vi "L298N_Driver.vi"() -> ()   [LabVIEW 2019]
uses:
  Commande 2.ctl
  <vilib>/myRIO/Instrument Drivers/Onboard IO/DIO/typedefs/DIO Reference.ctl
  <vilib>/myRIO/Common/Instrument Driver Framework/Utilities/typedefs/myRIO Generic Hardware Reference.ctl
  <vilib>/myRIO/Common/Instrument Driver Framework/Utilities/typedefs/Hardware Version Enum.ctl
  <vilib>/myRIO/Common/Instrument Driver Framework/Utilities/typedefs/myRIO v1.0 Reference.ctl
  <vilib>/myRIO/Common/Instrument Driver Framework/Utilities/typedefs/Generic FPGA Reference.ctl
  <vilib>/myRIO/Common/Instrument Driver Framework/myRIO v1.0/DIO/typedefs/DIO Channels List.ctl
  <vilib>/myRIO/Common/Instrument Driver Framework/myRIO v1.0/DIO/typedefs/DIO Channels Enum.ctl
  <vilib>/userDefined/High Color/nirio_resource_hc.ctl
  <vilib>/myRIO/Common/Instrument Driver Framework/myRIO v1.0/DIO/vis/myRIO v1.1 Open DIO.vi
  <vilib>/myRIO/Common/Instrument Driver Framework/Utilities/vis/Validate Channels.vi
  <vilib>/myRIO/Common/Instrument Driver Framework/myRIO v1.0/DIO/vis/myRIO v1.0 Reserve DIO.vi
  <vilib>/myRIO/Common/Instrument Driver Framework/myRIO v1.0/DIO/vis/myRIO v1.0 Close DIO.vi
  <vilib>/myRIO/Common/Instrument Driver Framework/myRIO v1.0/Resource Manager/vis/myRIO v1.0 Reserve Channel List.vi
  <vilib>/myRIO/Common/Instrument Driver Framework/myRIO v1.0/DIO/vis/myRIO v1.0 Build MUX Configuration DIO.vi
  <vilib>/myRIO/Common/Instrument Driver Framework/myRIO v1.0/DIO/vis/myRIO v1.0 Unreserve DIO.vi
  <vilib>/myRIO/Common/Instrument Driver Framework/myRIO v1.0/Resource Manager/vis/myRIO v1.0 Reserve Channel.vi
  <vilib>/myRIO/Common/Instrument Driver Framework/myRIO v1.0/Resource Manager/vis/myRIO v1.0 Unreserve Channel.vi
  <vilib>/myRIO/Common/Instrument Driver Framework/myRIO v1.0/Resource Manager/vis/myRIO v1.0 Create Configuration List.vi
  <vilib>/myRIO/Common/Instrument Driver Framework/myRIO v1.0/Resource Manager/vis/myRIO v1.0 Unreserve Channel List.vi
  <vilib>/myRIO/Common/Instrument Driver Framework/myRIO v1.0/Resource Manager/vis/myRIO v1.0 Build Mutex Name.vi
  <vilib>/Utility/VariantDataType/GetNumericInfo.vi
  <vilib>/Utility/error.llb/Error Cluster From Error Code.vi
  <vilib>/myRIO/Common/Instrument Driver Framework/myRIO v1.0/myRIO v1.1 Open.vi
  <vilib>/myRIO/Common/Instrument Driver Framework/Utilities/vis/IO Manager.vi
  <vilib>/myRIO/Common/Instrument Driver Framework/Utilities/vis/Configuration Manager.vi
  <vilib>/myRIO/Common/Instrument Driver Framework/myRIO v1.0/Resource Manager/vis/myRIO v1.0 Configure IO.vi
  <vilib>/myRIO/Common/Instrument Driver Framework/myRIO v1.0/myRIO v1.0 Close.vi
  <vilib>/myRIO/Common/Instrument Driver Framework/myRIO v1.0/DIO/vis/myRIO v1.0 Write DIO.vi
  <vilib>/myRIO/Common/Instrument Driver Framework/myRIO v1.0/DIO/vis/myRIO v1.0 Shutdown DIO.vi
  <vilib>/myRIO/Instrument Drivers/Onboard IO/DIO/vis/myRIO DIO Open.xnode
  <vilib>/myRIO/Instrument Drivers/Onboard IO/DIO/DIO.lvlib
panel:
  in  "Bouton Stop":bool
  out "Var_Etat":T1
  in  "PF_0":bool
  in  "PF_3":bool
  in  "PF_2":bool
  in  "PF_1":bool
  in  "PO_0":bool
  in  "PO_3":bool
  in  "PO_2":bool
  in  "PO_1":bool
  out "Moteur Porte 3":bool
  out "Moteur Porte 2":bool
  out "Moteur Porte 1":bool
  out "Moteur Porte 0":bool
  out "Moteur Cabine":bool
  in  "P0":bool
  in  "P3":bool
  in  "P2":bool
  in  "P1":bool
  in  "Etat_Asc":T1
  in  "Dest_3":bool
  in  "Dest_2":bool
  in  "Dest_1":bool
  in  "Dest_0":bool
  in  "Appel_0":bool
  in  "Appel_3":bool
  in  "Appel_2":bool
  in  "Appel_1":bool
  out "Cluster":T2
  in  "Énum":T3(ring)
  out "Etat":string
  out "Etat Ouvrir Porte 1":bool
  in  "Ouvrir Porte 1":bool
  out "error out 4":errorcluster caption="error out"
  in  "error in (no error) 4":errorcluster caption="error in (no error)"
  in  "Fermer  Porte 1":bool
  out "error out 3":errorcluster caption="error out"
  in  "error in (no error) 3":errorcluster caption="error in (no error)"
  out "error out 2":errorcluster caption="error out"
  in  "error in (no error) 2":errorcluster caption="error in (no error)"
  in  "Cabine Descendre":bool
  out "error out":errorcluster
  in  "error in (no error)":errorcluster
  in  "Cabine Monter":bool
  # "Simulation de présence cabine"
  # "Simulation de portes"
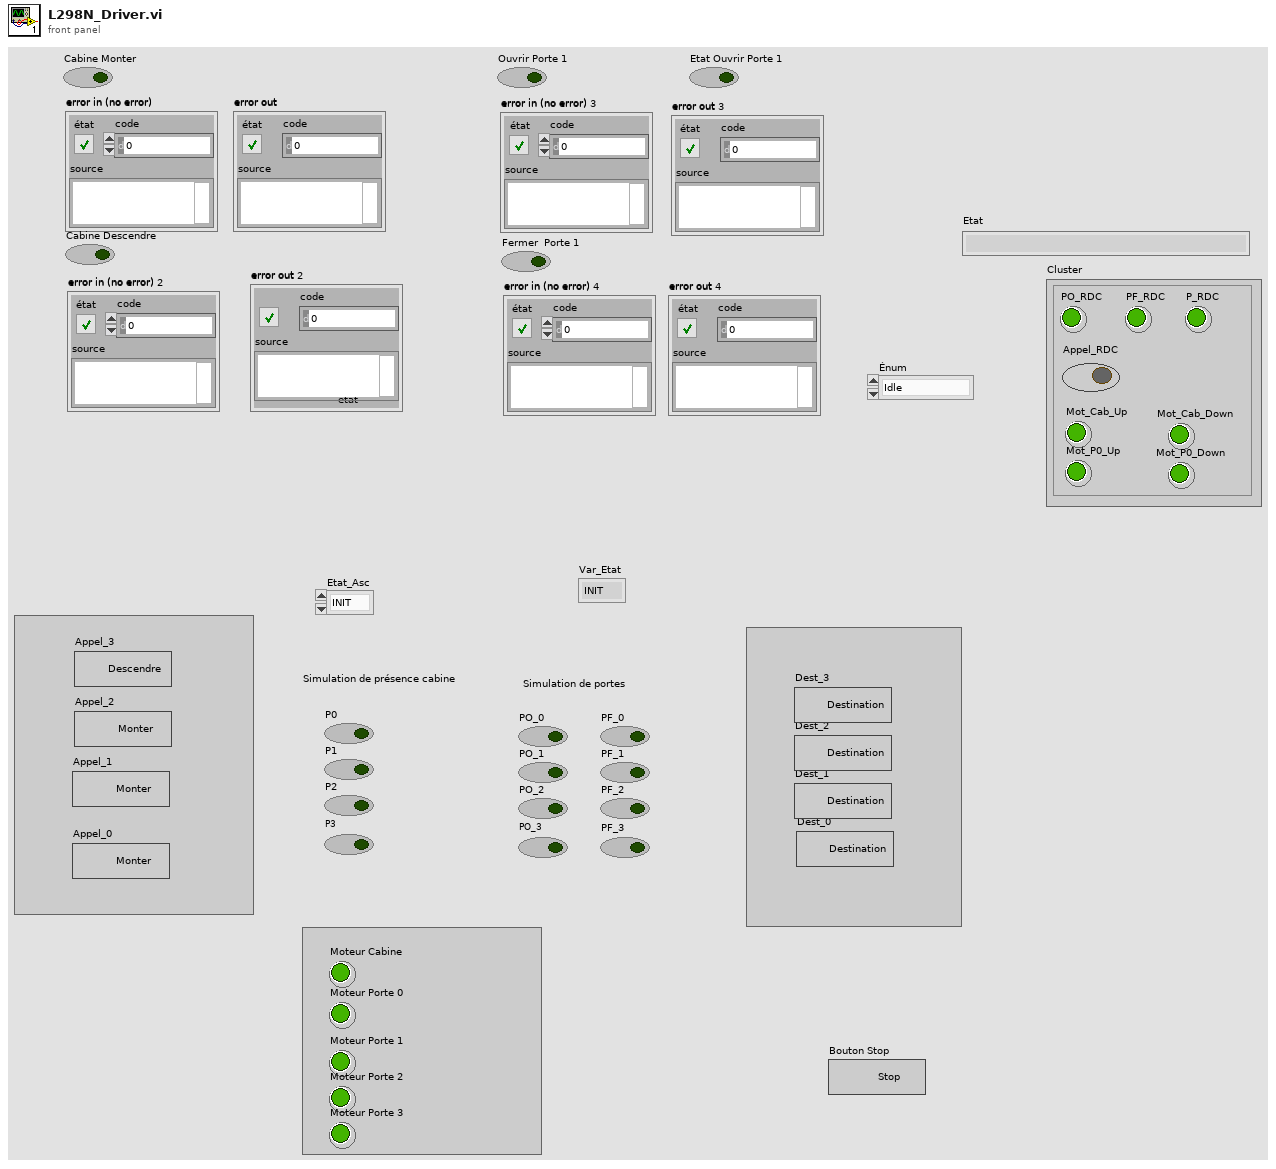
[diagram p1: front panel]
types:
  T1 = typedef "Commande 2.ctl" = enum16{"INIT", "REPOS", "DEPLACEMENT", "OUVERTURE_PORTE", "ATTENTE_TEMPO", "FERMETURE_PORTE", "ARRET_URGENCE"}
  T2 = cluster{"PO_RDC":bool, "PF_RDC":bool, "P_RDC":bool, "Appel_RDC":bool, "Mot_Cab_Up":bool, "Mot_Cab_Down":bool, "Mot_P0_Up":bool, "Mot_P0_Down":bool}
  T3 = enum16{"Idle", "Appel_Etage0", "Descente_Cabine", "Arrivee_Etage0", "Ouverture_Porte", "Attente_Porte", "Fermerture_Porte", "Fin", ""}
  T4 = typedef "DIO.lvlib/DIO Reference.ctl" = cluster{"myRIO Reference":T5, "DIO Channels List":T9}
  T5 = typedef "myRIO Generic Hardware Reference.ctl" = cluster{"myRIO Model":T6, "myRIO Hardware Reference":T7}
  T6 = typedef "Hardware Version Enum.ctl" = enum16{"Unknown", "myRIO-1900", "myRIO-1950", "roboRIO", "NI ELVIS RIO CM", "ELVIS III"}
  T7 = typedef "myRIO v1.0 Reference.ctl" = cluster{"Generic FPGA Reference":T8, "Allow multiple opens":bool}
  T8 = typedef "Generic FPGA Reference.ctl" = refnum<k20>
  T9 = typedef "DIO Channels List.ctl" = T10[]
  T10 = typedef "DIO Channels Enum.ctl" = enum16{"Not Connected", "C/DIO0", "C/DIO1", "C/DIO2", "C/DIO3", "C/DIO4", "C/DIO5", "C/DIO6", "C/DIO7", "A/DIO0", "A/DIO1", "A/DIO2", "A/DIO3", "A/DIO4", "A/DIO5", "A/DIO6", "A/DIO7", "A/DIO8", "A/DIO9", "A/DIO10", "A/DIO11", "A/DIO12", "A/DIO13", "A/DIO14", "A/DIO15", "A/DIO16", "A/DIO17", "A/DIO18", "A/DIO19", "B/DIO0", "B/DIO1", "B/DIO2", "B/DIO3", "B/DIO4", "B/DIO5", "B/DIO6", "B/DIO7", "B/DIO8", "B/DIO9", "B/DIO10", "B/DIO11", "B/DIO12", "B/DIO13", "B/DIO14", "B/DIO15", "B/DIO16", "B/DIO17", "B/DIO18", "B/DIO19", "LED0", "LED1", "LED2", "LED3", "Button0", "DIO/DIO0", "DIO/DIO1", "DIO/DIO2", "DIO/DIO3", "DIO/DIO4", "DIO/DIO5", "DIO/DIO6", "DIO/DIO7", "DIO/DIO8", "DIO/DIO9", "SPI/CS0", "SPI/CS1", "SPI/CS2", "SPI/CS3", "LED RADIO (Green)", "LED RADIO (Red)", "LED COMM (Green)", "LED COMM (Red)", "LED MODE (Green)", "LED MODE (Red)"}
  T11 = typedef "nirio_resource_hc.ctl" = tag
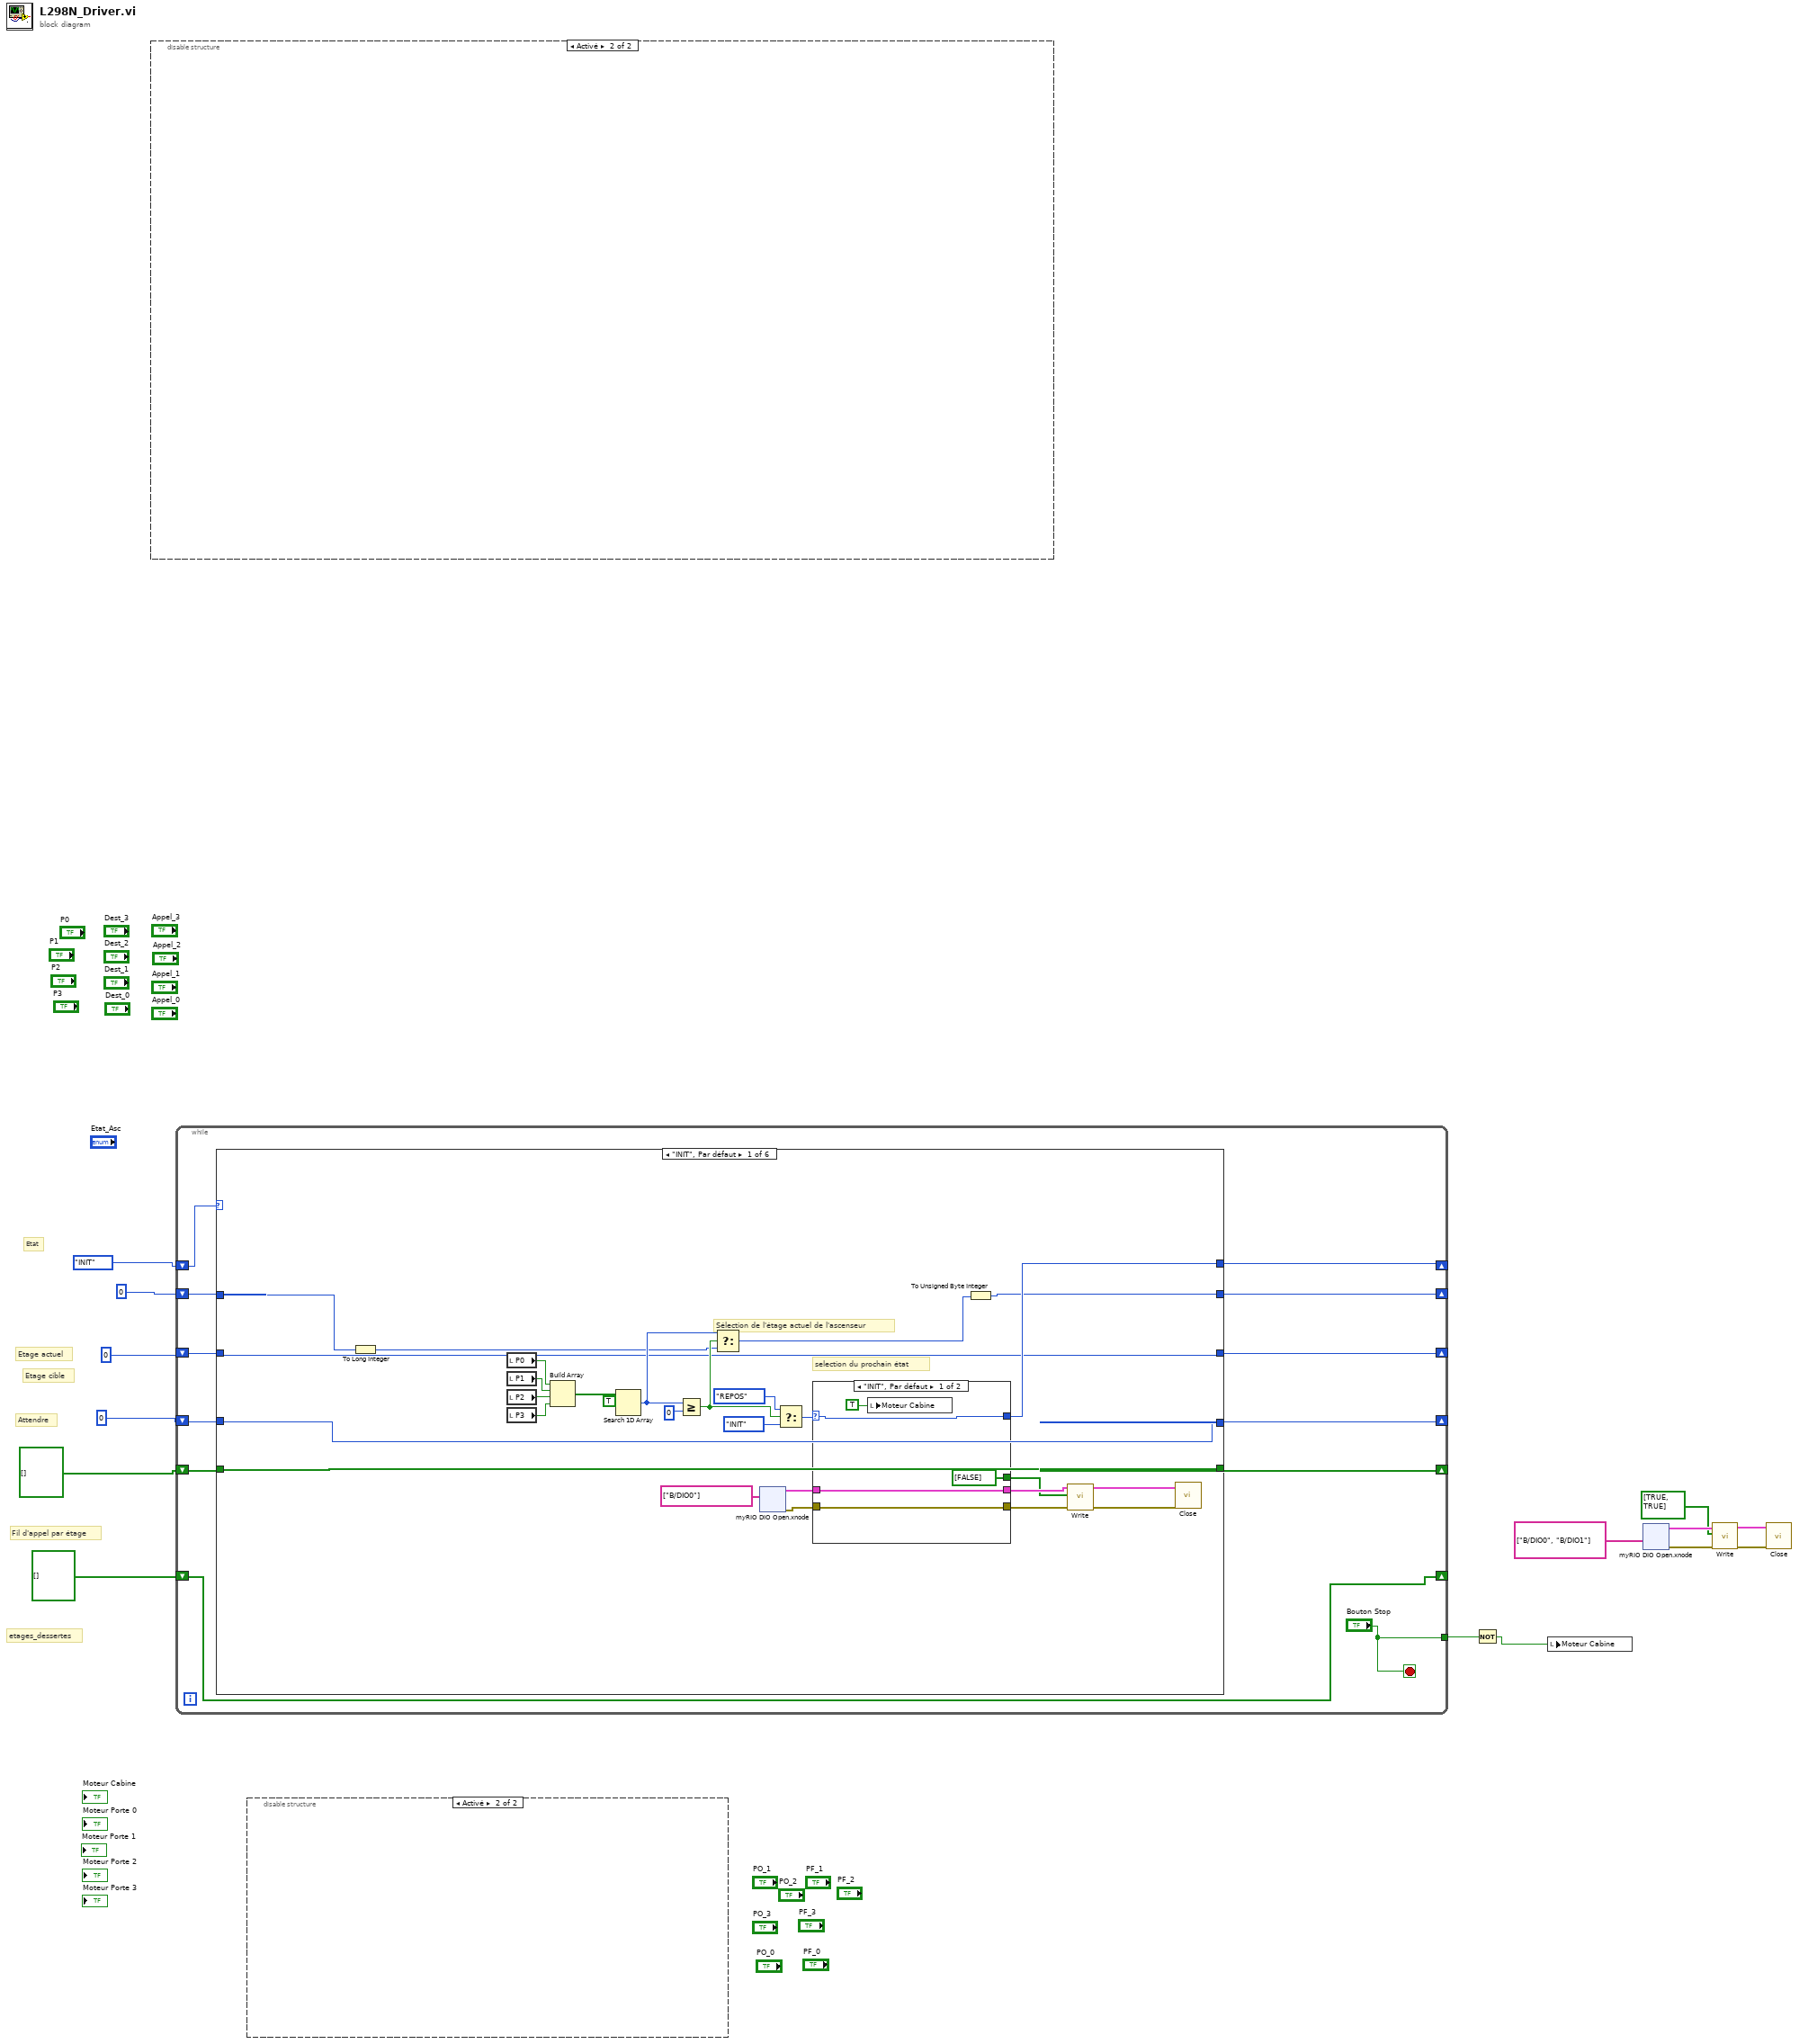
[diagram p0: block diagram]
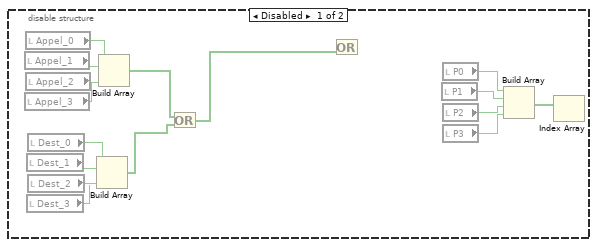
[diagram p2: hidden frame]
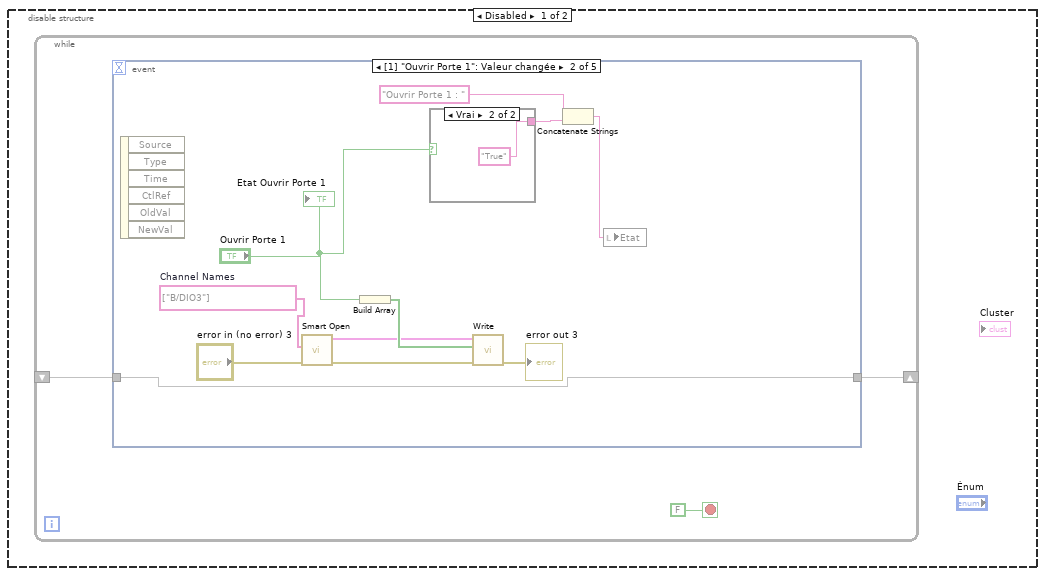
[diagram p3: hidden frame]
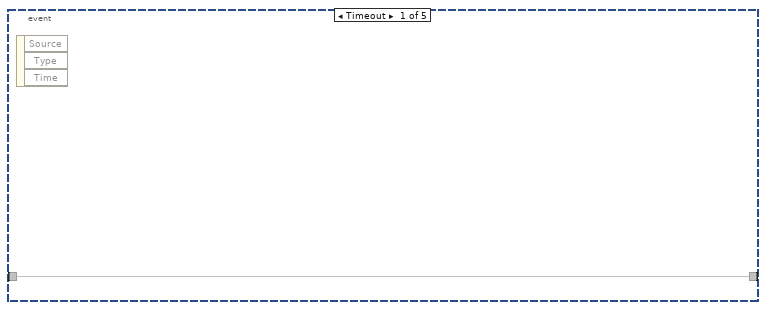
[diagram p4: hidden frame]
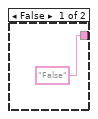
[diagram p5: hidden frame]
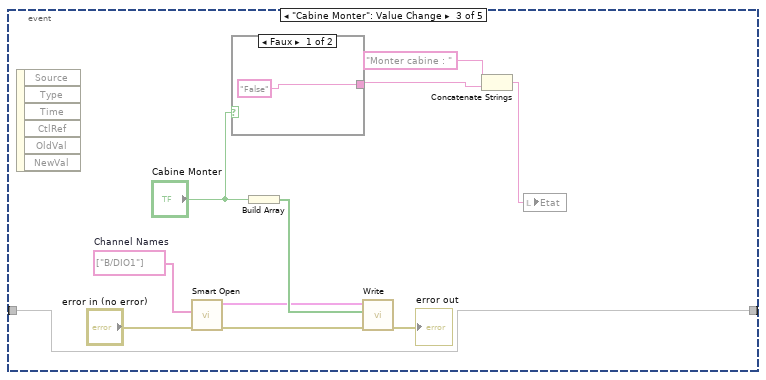
[diagram p6: hidden frame]
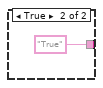
[diagram p7: hidden frame]
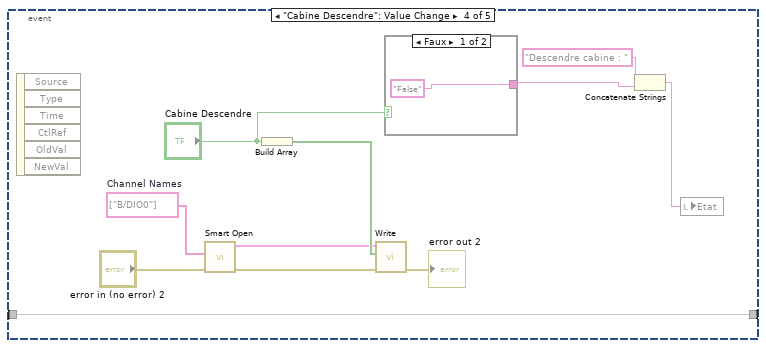
[diagram p8: hidden frame]
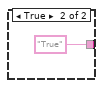
[diagram p9: hidden frame]
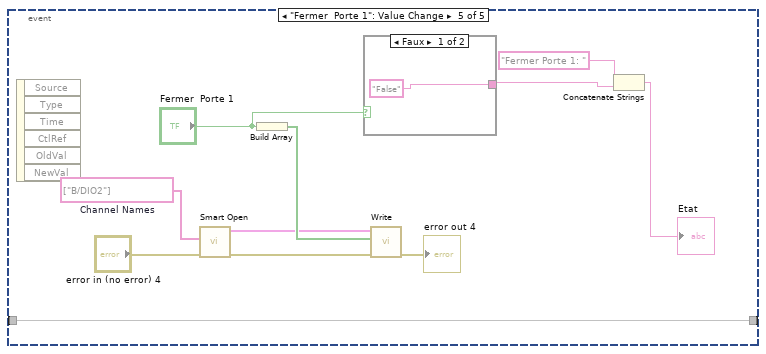
[diagram p10: hidden frame]
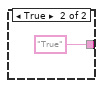
[diagram p11: hidden frame]
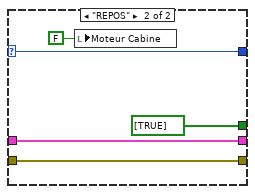
[diagram p12: hidden frame]
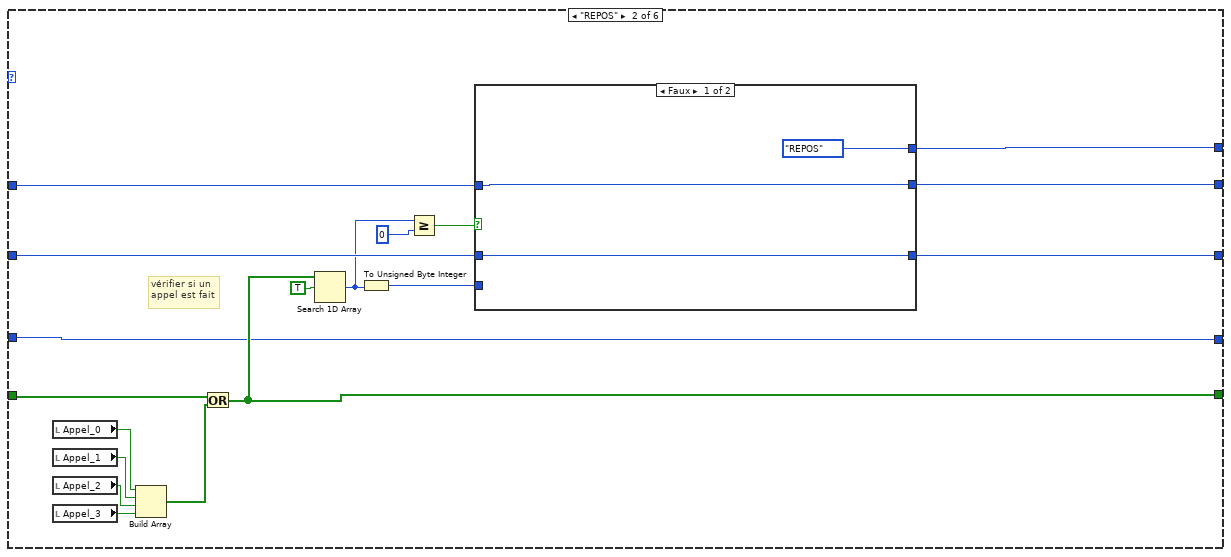
[diagram p13: hidden frame]
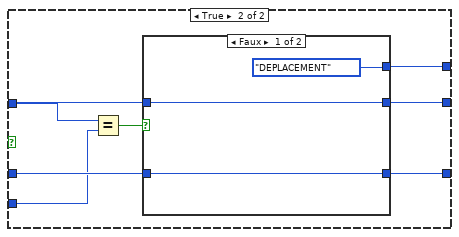
[diagram p14: hidden frame]
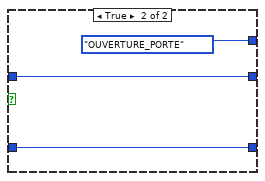
[diagram p15: hidden frame]
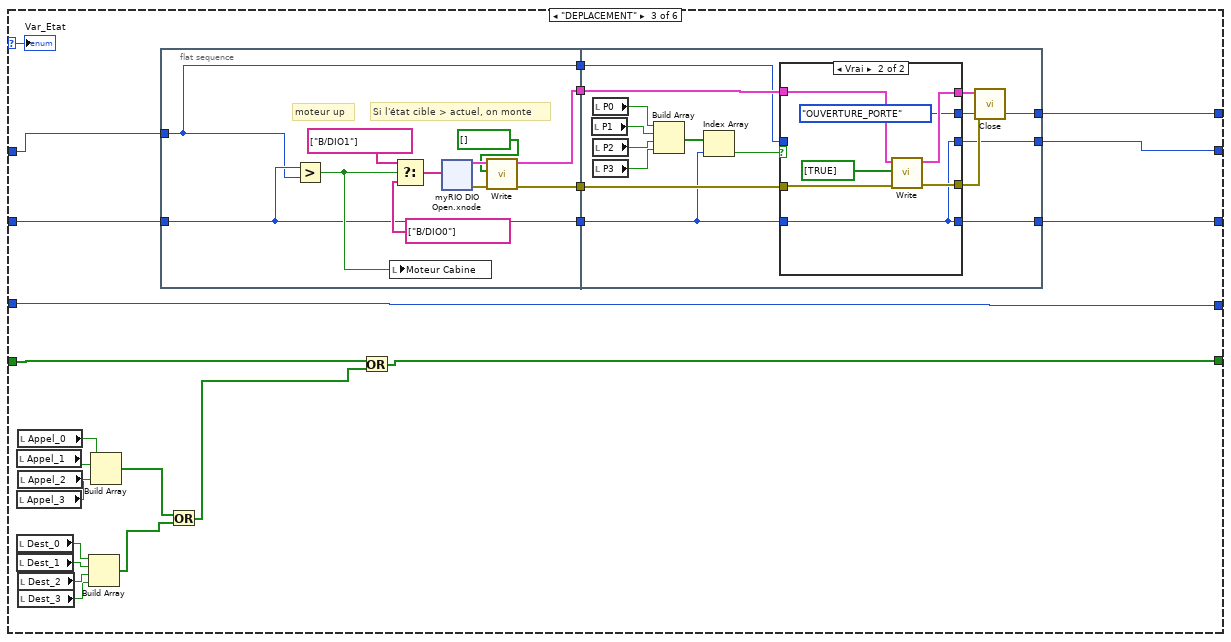
[diagram p16: hidden frame]
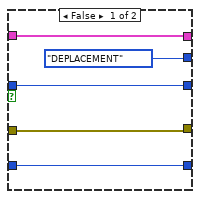
[diagram p17: hidden frame]
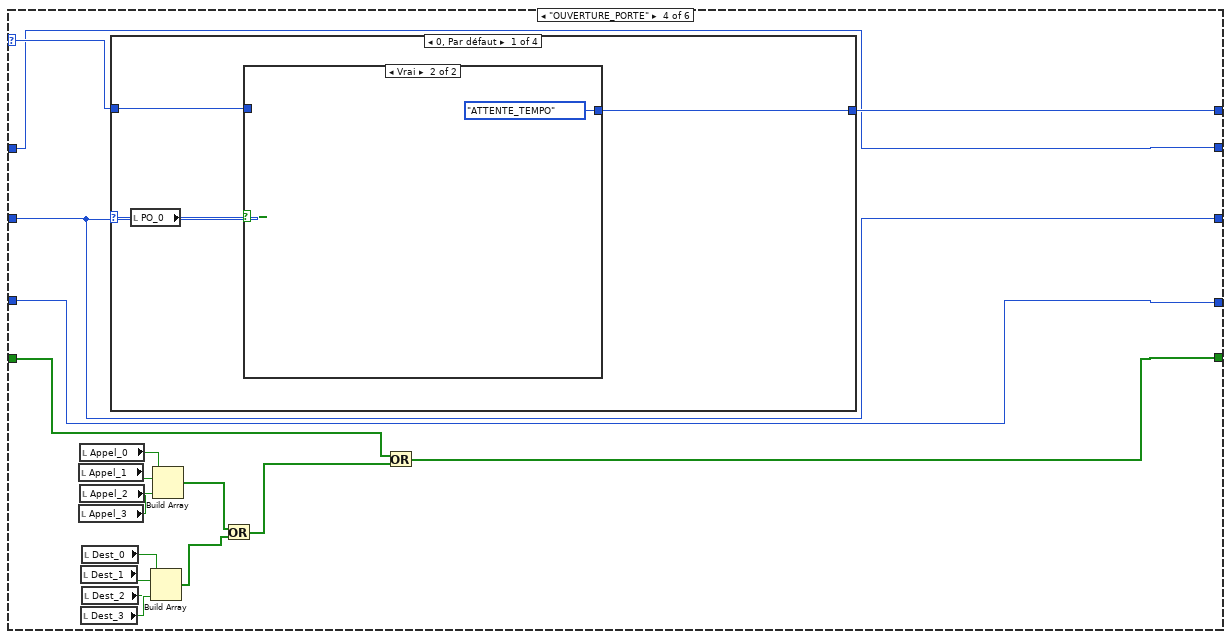
[diagram p18: hidden frame]
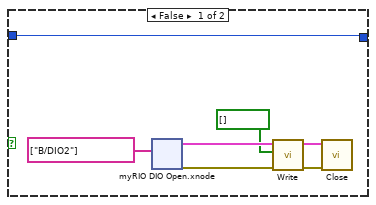
[diagram p19: hidden frame]
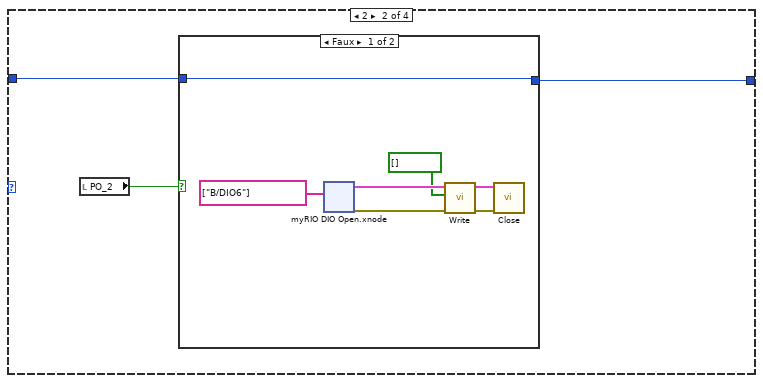
[diagram p20: hidden frame]
diagram:
  # "etages_dessertes"
  # "Fil d'appel par étage"
  # "Attendre"
  # "Etage cible"
  # "Etage actuel"
  # "Etat"
  n1 = disable-structure shown="Activé" {
    frame Disabled {
      n2 = while {
        shift-right: [w15] -> _
        shift-left: _ -> [w16]
        stop <- FALSE stop-if-true
        n3 = event shown="[1] \"Ouvrir Porte 1\": Valeur changée" {
          selector: _ -> [_ _ _ _ _]
          dyn-events: _ -> [_ _ _ _ _]
          timeout: _ -> [_ _ _ _ _]
          tunnel: [w18 w19 w32 w45 w58] -> w15
          tunnel: w16 -> [w18 w19 w32 w45 w58]
          event Timeout {
            n4 = event-data() -> ()  [unwired: 1 in, 3 out]
          }
          event "Ouvrir Porte 1": Value Change {
            w25 = tag[] ["B/DIO3"]  # Channel Names
            n5 = event-data() -> ()  [unwired: 1 in, 6 out]
            n6 = call <vilib>:"Smart Open.vi"("error in (no error)"="error in (no error) 3", "Channel Names"=w25) -> ("error out"=w26:errorcluster, "DIO Ref Out"=w27:T4)  [unwired: 8 in]
            n7 = Build Array("Ouvrir Porte 1") -> (w29:bool[])
            n8 = case shown="Vrai" "Ouvrir Porte 1" {
              tunnel: ["False" "True"] -> w21
              frame False {
              }
              frame True {
              }
            }
            n9 = call <vilib>:"Write.vi"("error in (no error)"=w26, "Values"=w29, "DIO Ref In"=w27) -> ("error out"=→"error out 3":errorcluster)  [unwired: 6 in, 1 out]
            n10 = Concatenate Strings("Ouvrir Porte 1 : " ("chaîne"), w21) -> (w20:string)
            n11 = local write "Etat"(w20) -> ()
            "Etat Ouvrir Porte 1" <- "Ouvrir Porte 1"
          }
          event "Cabine Monter": Value Change {
            w37 = tag[] ["B/DIO1"]  # Channel Names
            n12 = event-data() -> ()  [unwired: 1 in, 6 out]
            n13 = call <vilib>:"Smart Open.vi"("error in (no error)"="error in (no error)", "Channel Names"=w37) -> ("error out"=w39:errorcluster, "DIO Ref Out"=w40:T4)  [unwired: 8 in]
            n14 = case shown="Faux" "Cabine Monter" {
              tunnel: ["False" "True"] -> w35
              frame False {
              }
              frame True {
              }
            }
            n15 = Build Array("Cabine Monter") -> (w42:bool[])
            n16 = call <vilib>:"Write.vi"("error in (no error)"=w39, "Values"=w42, "DIO Ref In"=w40) -> ("error out"=→"error out":errorcluster)  [unwired: 6 in, 1 out]
            n17 = Concatenate Strings("Monter cabine : " ("chaîne"), w35) -> (w34:string)
            n18 = local write "Etat"(w34) -> ()
          }
          event "Cabine Descendre": Value Change {
            w50 = tag[] ["B/DIO0"]  # Channel Names
            n19 = event-data() -> ()  [unwired: 1 in, 6 out]
            n20 = call <vilib>:"Smart Open.vi"("error in (no error)"="error in (no error) 2", "Channel Names"=w50) -> ("error out"=w52:errorcluster, "DIO Ref Out"=w53:T4)  [unwired: 8 in]
            n21 = Build Array("Cabine Descendre") -> (w55:bool[])
            n22 = call <vilib>:"Write.vi"("error in (no error)"=w52, "Values"=w55, "DIO Ref In"=w53) -> ("error out"=→"error out 2":errorcluster)  [unwired: 6 in, 1 out]
            n23 = case shown="Faux" "Cabine Descendre" {
              tunnel: ["False" "True"] -> w48
              frame False {
              }
              frame True {
              }
            }
            n24 = Concatenate Strings("Descendre cabine : " ("chaîne"), w48) -> (w47:string)
            n25 = local write "Etat"(w47) -> ()
          }
          event "Fermer  Porte 1": Value Change {
            w63 = tag[] ["B/DIO2"]  # Channel Names
            n26 = event-data() -> ()  [unwired: 1 in, 6 out]
            n27 = call <vilib>:"Smart Open.vi"("error in (no error)"="error in (no error) 4", "Channel Names"=w63) -> ("error out"=w65:errorcluster, "DIO Ref Out"=w66:T4)  [unwired: 8 in]
            n28 = Build Array("Fermer  Porte 1") -> (w68:bool[])
            n29 = case shown="Faux" "Fermer  Porte 1" {
              tunnel: ["False" "True"] -> w61
              frame False {
              }
              frame True {
              }
            }
            n30 = call <vilib>:"Write.vi"("error in (no error)"=w65, "Values"=w68, "DIO Ref In"=w66) -> ("error out"=→"error out 4":errorcluster)  [unwired: 6 in, 1 out]
            n31 = Concatenate Strings("Fermer Porte 1: " ("chaîne"), w61) -> (→"Etat":string)
          }
        }
      }
    }
    frame Enabled {
    }
  }
  n32 = while {
    shift-right: [w75] -> _
    shift-left: Commande_2."INIT" ("Etat_Asc") -> [w82]
    shift-right: [w76] -> _
    shift-left: u8 0 -> [w81]
    shift-right: [w77] -> _
    shift-left: u8 0 -> [w80]
    shift-right: [w73] -> _
    shift-left: 0 -> [w79]
    shift-right: [w74] -> _
    shift-left: bool[] [] -> [w78]
    shift-right: [w72] -> _
    shift-left: bool[] [] -> [w72]
    tunnel: ["Bouton Stop"] -> w2
    stop <- "Bouton Stop" stop-if-true
    n33 = case shown="\"INIT\", Par défaut" w82 {
      selector: w82 -> [_ _ w171 w266 _ w396]
      tunnel: w81 -> [w102 w139 w188 w264 w391 w397]
      tunnel: [w100 w150 w178 w265 Commande_2."FERMETURE_PORTE" ("Etat_Asc") w395] -> w75
      tunnel: w80 -> [w99 w148 w189 w263 w390 w394]
      tunnel: [w99 w149 w186 w263 w390 w394] -> w77
      tunnel: w79 -> [w83 w137 w190 w262 w389 w393]
      tunnel: [w98 w145 w179 w249 w375 w398] -> w74
      tunnel: w78 -> [w98 w147 w180 w250 w376 w399]
      tunnel: [w84 w138 w176 w264 w391 w397] -> w76
      tunnel: [w83 w137 w190 w262 w389 w393] -> w73
      frame "INIT", Default {
        # "Sélection de l'étage actuel de l'ascenseur"
        # "selection du prochain état"
        n34 = To Long Integer(number=w102) -> (32bit integer=w103:i32)
        n35 = local read "P0"() -> (w97:bool)
        n36 = local read "P1"() -> (w96:bool)
        n37 = local read "P2"() -> (w95:bool)
        n38 = local read "P3"() -> (w94:bool)
        n39 = Build Array(w97, w96, w95, w94) -> (w110:bool[])
        n40 = Search 1D Array(1D array=w110, element=TRUE ("élément")) -> (index of element=w104:i32)  [unwired: 1 in]
        n41 = Greater Or Equal?(x=w104, y=0) -> (x >= y?=w105:bool)
        n42 = Select(t=w104, s=w105, f=w103) -> (s? t:f=w85:i32)
        n43 = xnode "myRIO DIO Open.xnode"("Channel Names"=tag[] ["B/DIO0"]) -> ("error out"=w91:errorcluster, "DIO Ref Out"=w92:T4)  [unwired: 2 in]
        n44 = Select(t=Commande_2."REPOS" ("Etat_Asc"), s=w105, f=Commande_2."INIT" ("Etat_Asc")) -> (s? t:f=w101:T1)
        n45 = case shown="\"INIT\", Par défaut" w101 {
          selector: w101 -> [w130 w136]
          tunnel: [w130 w136] -> w100
          tunnel: w92 -> [w129 w134]
          tunnel: w91 -> [w128 w133]
          tunnel: [w129 w134] -> w90
          tunnel: [w128 w133] -> w89
          tunnel: [bool[] [FALSE] ("Values") bool[] [TRUE] ("Values")] -> w86
          frame "INIT", Default {
            n46 = local write "Moteur Cabine"(TRUE ("Moteur Cabine")) -> ()
          }
          frame "REPOS" {
            n47 = local write "Moteur Cabine"(FALSE ("Moteur Cabine")) -> ()
          }
        }
        n48 = To Unsigned Byte Integer(number=w85) -> (unsigned 8bit integer=w84:u8)
        n49 = call <vilib>:"Write.vi"("error in (no error)"=w89, "Values"=w86, "DIO Ref In"=w90) -> ("error out"=w88:errorcluster, "DIO Ref Out"=w87:T4)  [unwired: 6 in]
        n50 = call <vilib>:"Close.vi"("error in (no error)"=w88, "DIO Ref In"=w87) -> ()  [unwired: 9 in, 1 out]
      }
      frame "REPOS" {
        # "vérifier si un appel est fait"
        n51 = local read "Appel_0"() -> (w154:bool)
        n52 = local read "Appel_1"() -> (w153:bool)
        n53 = local read "Appel_2"() -> (w152:bool)
        n54 = local read "Appel_3"() -> (w151:bool)
        n55 = Build Array(w154, w153, w152, w151) -> (w146:bool[])
        n56 = Or(x=w147, y=w146) -> (x .or. y?=w145:bool[])
        n57 = Search 1D Array(1D array=w145, element=TRUE ("élément")) -> (index of element=w143:i32)  [unwired: 1 in]
        n58 = To Unsigned Byte Integer(number=w143) -> (unsigned 8bit integer=w140:u8)
        n59 = Greater Or Equal?(x=w143, y=0) -> (x >= y?=w141:bool)
        n60 = case shown="Faux" w141 {
          tunnel: [Commande_2."REPOS" ("Etat_Asc") w163] -> w150
          tunnel: [w156 w162] -> w149
          tunnel: w148 -> [w156 w161]
          tunnel: w140 -> [_ w160]
          tunnel: w139 -> [w155 w158]
          tunnel: [w155 w159] -> w138
          frame False {
          }
          frame True {
            n61 = Equal?(x=w158, y=w160) -> (x = y?=w164:bool)
            n62 = case shown="Faux" w164 {
              tunnel: [Commande_2."DEPLACEMENT" ("Etat_Asc") Commande_2."OUVERTURE_PORTE" ("Etat_Asc")] -> w163
              tunnel: [w165 w169] -> w162
              tunnel: w161 -> [w165 w169]
              tunnel: w158 -> [w166 w168]
              tunnel: [w166 w168] -> w159
              frame False {
              }
              frame True {
              }
            }
          }
        }
      }
      frame "DEPLACEMENT" {
        n63 = local read "Appel_1"() -> (w193:bool)
        n64 = local read "Appel_3"() -> (w191:bool)
        n65 = local read "Dest_0"() -> (w175:bool)
        n66 = local read "Dest_1"() -> (w174:bool)
        n67 = local read "Appel_0"() -> (w194:bool)
        n68 = local read "Appel_2"() -> (w192:bool)
        n69 = local read "Dest_2"() -> (w173:bool)
        n70 = local read "Dest_3"() -> (w172:bool)
        n71 = Build Array(w175, w174, w173, w172) -> (w182:bool[])
        n72 = Build Array(w194, w193, w192, w191) -> (w183:bool[])
        n73 = flat-sequence {
          tunnel: w188 -> [w195]
          tunnel: w189 -> [w198]
          tunnel: [w198] -> w187
          tunnel: [w197] -> w185
          tunnel: [w196] -> w184
          tunnel: [w195] -> w177
          tunnel: w187 -> [w222]
          tunnel: [w223] -> w186
          tunnel: w185 -> [w230]
          tunnel: w184 -> [w228]
          tunnel: [w226] -> w178
          tunnel: w177 -> [w225]
          tunnel: [w224] -> w176
          frame #0 {
            # "Si l'état cible > actuel, on monte"
            # "moteur up"
            n74 = Greater?(x=w198, y=w195) -> (0:w199:bool)
            n75 = local write "Moteur Cabine"(w199) -> ()
            n76 = Select(t=tag[] ["B/DIO1"] ("Channel Names"), s=w199, f=tag[] ["B/DIO0"] ("Channel Names")) -> (s? t:f=w203:tag[])
            n77 = xnode "myRIO DIO Open.xnode"("Channel Names"=w203) -> ("error out"=w205:errorcluster, "DIO Ref Out"=w204:T4)  [unwired: 2 in]
            n78 = call <vilib>:"Write.vi"("error in (no error)"=w205, "Values"=bool[] [], "DIO Ref In"=w204) -> ("error out"=w197:errorcluster, "DIO Ref Out"=w196:T4)  [unwired: 6 in]
          }
          frame #1 {
            n79 = local read "P1"() -> (w235:bool)
            n80 = local read "P0"() -> (w236:bool)
            n81 = local read "P2"() -> (w234:bool)
            n82 = local read "P3"() -> (w233:bool)
            n83 = Build Array(w236, w235, w234, w233) -> (w232:bool[])
            n84 = Index Array(array=w232, index=w222) -> (element=w231:bool)
            n85 = case shown="Vrai" w231 {
              tunnel: [w241 w247] -> w229
              tunnel: w230 -> [w241 w246]
              tunnel: w228 -> [w240 w244]
              tunnel: [w240 w248] -> w227
              tunnel: [Commande_2."DEPLACEMENT" ("Etat_Asc") Commande_2."OUVERTURE_PORTE" ("Etat_Asc")] -> w226
              tunnel: w225 -> [w238 _]
              tunnel: [w238 w242] -> w224
              tunnel: [w237 w242] -> w223
              tunnel: w222 -> [w237 w242]
              frame False {
              }
              frame True {
                n86 = call <vilib>:"Write.vi"("error in (no error)"=w246, "Values"=bool[] [TRUE], "DIO Ref In"=w244) -> ("error out"=w247:errorcluster, "DIO Ref Out"=w248:T4)  [unwired: 6 in]
              }
            }
            n87 = call <vilib>:"Close.vi"("error in (no error)"=w229, "DIO Ref In"=w227) -> ()  [unwired: 9 in, 1 out]
          }
        }
        n88 = Or(x=w183, y=w182) -> (x .or. y?=w181:bool[])
        n89 = Or(x=w180, y=w181) -> (x .or. y?=w179:bool[])
        "Var_Etat" <- w171
      }
      frame "OUVERTURE_PORTE" {
        n90 = local read "Appel_1"() -> (w260:bool)
        n91 = local read "Appel_3"() -> (w258:bool)
        n92 = local read "Appel_0"() -> (w261:bool)
        n93 = local read "Appel_2"() -> (w259:bool)
        n94 = local read "Dest_1"() -> (w255:bool)
        n95 = local read "Dest_3"() -> (w257:bool)
        n96 = local read "Dest_0"() -> (w254:bool)
        n97 = local read "Dest_2"() -> (w256:bool)
        n98 = case shown="0, Par défaut" w263 {
          tunnel: w266 -> [w267 w295 w321 w348]
          tunnel: [w268 w296 w322 w349] -> w265
          frame 0, Default {
            n99 = local read "PO_0"() -> (w269:bool)
            n100 = case shown="Vrai" w269 {
              tunnel: w267 -> [w276 _]
              tunnel: [w276 Commande_2."ATTENTE_TEMPO" ("Etat_Asc")] -> w268
              frame False {
                n101 = xnode "myRIO DIO Open.xnode"("Channel Names"=tag[] ["B/DIO2"]) -> ("error out"=w273:errorcluster, "DIO Ref Out"=w272:T4)  [unwired: 2 in]
                n102 = call <vilib>:"Write.vi"("error in (no error)"=w273, "Values"=bool[] [], "DIO Ref In"=w272) -> ("error out"=w274:errorcluster, "DIO Ref Out"=w275:T4)  [unwired: 6 in]
                n103 = call <vilib>:"Close.vi"("error in (no error)"=w274, "DIO Ref In"=w275) -> ()  [unwired: 9 in, 1 out]
              }
              frame True {
              }
            }
          }
          frame 2 {
            n104 = local read "PO_2"() -> (w294:bool)
            n105 = case shown="Faux" w294 {
              tunnel: w295 -> [w303 _]
              tunnel: [w303 Commande_2."ATTENTE_TEMPO" ("Etat_Asc")] -> w296
              frame False {
                n106 = xnode "myRIO DIO Open.xnode"("Channel Names"=tag[] ["B/DIO6"]) -> ("error out"=w300:errorcluster, "DIO Ref Out"=w299:T4)  [unwired: 2 in]
                n107 = call <vilib>:"Write.vi"("error in (no error)"=w300, "Values"=bool[] [], "DIO Ref In"=w299) -> ("error out"=w301:errorcluster, "DIO Ref Out"=w302:T4)  [unwired: 6 in]
                n108 = call <vilib>:"Close.vi"("error in (no error)"=w301, "DIO Ref In"=w302) -> ()  [unwired: 9 in, 1 out]
              }
              frame True {
              }
            }
          }
          frame 3 {
            n109 = local read "PO_3"() -> (w323:bool)
            n110 = case shown="Vrai" w323 {
              tunnel: [w324 Commande_2."ATTENTE_TEMPO" ("Etat_Asc")] -> w322
              tunnel: w321 -> [w324 _]
              frame False {
                n111 = xnode "myRIO DIO Open.xnode"("Channel Names"=tag[] ["B/DIO8"]) -> ("error out"=w328:errorcluster, "DIO Ref Out"=w327:T4)  [unwired: 2 in]
                n112 = call <vilib>:"Write.vi"("error in (no error)"=w328, "Values"=bool[] [], "DIO Ref In"=w327) -> ("error out"=w329:errorcluster, "DIO Ref Out"=w330:T4)  [unwired: 6 in]
                n113 = call <vilib>:"Close.vi"("error in (no error)"=w329, "DIO Ref In"=w330) -> ()  [unwired: 9 in, 1 out]
              }
              frame True {
              }
            }
          }
          frame 1 {
            n114 = local read "PO_1"() -> (w350:bool)
            n115 = case shown="Vrai" w350 {
              tunnel: [w351 Commande_2."ATTENTE_TEMPO" ("Etat_Asc")] -> w349
              tunnel: w348 -> [w351 _]
              frame False {
                n116 = xnode "myRIO DIO Open.xnode"("Channel Names"=tag[] ["B/DIO4"]) -> ("error out"=w355:errorcluster, "DIO Ref Out"=w354:T4)  [unwired: 2 in]
                n117 = call <vilib>:"Write.vi"("error in (no error)"=w355, "Values"=bool[] [], "DIO Ref In"=w354) -> ("error out"=w356:errorcluster, "DIO Ref Out"=w357:T4)  [unwired: 6 in]
                n118 = call <vilib>:"Close.vi"("error in (no error)"=w356, "DIO Ref In"=w357) -> ()  [unwired: 9 in, 1 out]
              }
              frame True {
              }
            }
          }
        }
        n119 = Build Array(w254, w255, w256, w257) -> (w252:bool[])
        n120 = Build Array(w261, w260, w259, w258) -> (w253:bool[])
        n121 = Or(x=w253, y=w252) -> (x .or. y?=w251:bool[])
        n122 = Or(x=w250, y=w251) -> (x .or. y?=w249:bool[])
      }
      frame "ATTENTE_TEMPO" {
        n123 = local read "Appel_1"() -> (w386:bool)
        n124 = local read "Appel_3"() -> (w384:bool)
        n125 = local read "Appel_0"() -> (w387:bool)
        n126 = local read "Appel_2"() -> (w385:bool)
        n127 = local read "Dest_1"() -> (w381:bool)
        n128 = local read "Dest_3"() -> (w383:bool)
        n129 = local read "Dest_0"() -> (w380:bool)
        n130 = local read "Dest_2"() -> (w382:bool)
        n131 = Build Array(w380, w381, w382, w383) -> (w378:bool[])
        n132 = Build Array(w387, w386, w385, w384) -> (w379:bool[])
        n133 = Or(x=w379, y=w378) -> (x .or. y?=w377:bool[])
        n134 = Or(x=w376, y=w377) -> (x .or. y?=w375:bool[])
        n135 = Wait (ms)(milliseconds to wait=u32 3000 ("attente (ms)")) -> ()  [unwired: 1 out]
      }
      frame "FERMETURE_PORTE" {
        n136 = local read "Appel_1"() -> (w409:bool)
        n137 = local read "Appel_3"() -> (w407:bool)
        n138 = local read "Appel_0"() -> (w410:bool)
        n139 = local read "Appel_2"() -> (w408:bool)
        n140 = Build Array(w410, w409, w408, w407) -> (w402:bool[])
        n141 = case shown="0, Par défaut" w394 {
          tunnel: w396 -> [w411 w439 w465 w492]
          tunnel: [w412 w440 w466 w493] -> w395
          frame 0, Default {
            n142 = local read "PO_0"() -> (w413:bool)
            n143 = case shown="Vrai" w413 {
              tunnel: w411 -> [w420 _]
              tunnel: [w420 Commande_2."REPOS" ("Etat_Asc")] -> w412
              frame False {
                n144 = xnode "myRIO DIO Open.xnode"("Channel Names"=tag[] ["B/DIO3"]) -> ("error out"=w417:errorcluster, "DIO Ref Out"=w416:T4)  [unwired: 2 in]
                n145 = call <vilib>:"Write.vi"("error in (no error)"=w417, "Values"=bool[] [], "DIO Ref In"=w416) -> ("error out"=w418:errorcluster, "DIO Ref Out"=w419:T4)  [unwired: 6 in]
                n146 = call <vilib>:"Close.vi"("error in (no error)"=w418, "DIO Ref In"=w419) -> ()  [unwired: 9 in, 1 out]
              }
              frame True {
              }
            }
          }
          frame 2 {
            n147 = local read "PO_2"() -> (w438:bool)
            n148 = case shown="Vrai" w438 {
              tunnel: w439 -> [w447 _]
              tunnel: [w447 Commande_2."REPOS" ("Etat_Asc")] -> w440
              frame False {
                n149 = xnode "myRIO DIO Open.xnode"("Channel Names"=tag[] ["B/DIO6"]) -> ("error out"=w444:errorcluster, "DIO Ref Out"=w443:T4)  [unwired: 2 in]
                n150 = call <vilib>:"Write.vi"("error in (no error)"=w444, "Values"=bool[] [], "DIO Ref In"=w443) -> ("error out"=w445:errorcluster, "DIO Ref Out"=w446:T4)  [unwired: 6 in]
                n151 = call <vilib>:"Close.vi"("error in (no error)"=w445, "DIO Ref In"=w446) -> ()  [unwired: 9 in, 1 out]
              }
              frame True {
              }
            }
          }
          frame 3 {
            n152 = local read "PO_3"() -> (w467:bool)
            n153 = case shown="Vrai" w467 {
              tunnel: [w468 Commande_2."REPOS" ("Etat_Asc")] -> w466
              tunnel: w465 -> [w468 _]
              frame False {
                n154 = xnode "myRIO DIO Open.xnode"("Channel Names"=tag[] ["B/DIO8"]) -> ("error out"=w472:errorcluster, "DIO Ref Out"=w471:T4)  [unwired: 2 in]
                n155 = call <vilib>:"Write.vi"("error in (no error)"=w472, "Values"=bool[] [], "DIO Ref In"=w471) -> ("error out"=w473:errorcluster, "DIO Ref Out"=w474:T4)  [unwired: 6 in]
                n156 = call <vilib>:"Close.vi"("error in (no error)"=w473, "DIO Ref In"=w474) -> ()  [unwired: 9 in, 1 out]
              }
              frame True {
              }
            }
          }
          frame 1 {
            n157 = local read "PO_1"() -> (w494:bool)
            n158 = case shown="Vrai" w494 {
              tunnel: [w495 Commande_2."REPOS" ("Etat_Asc")] -> w493
              tunnel: w492 -> [w495 _]
              frame False {
                n159 = xnode "myRIO DIO Open.xnode"("Channel Names"=tag[] ["B/DIO4"]) -> ("error out"=w499:errorcluster, "DIO Ref Out"=w498:T4)  [unwired: 2 in]
                n160 = call <vilib>:"Write.vi"("error in (no error)"=w499, "Values"=bool[] [], "DIO Ref In"=w498) -> ("error out"=w500:errorcluster, "DIO Ref Out"=w501:T4)  [unwired: 6 in]
                n161 = call <vilib>:"Close.vi"("error in (no error)"=w500, "DIO Ref In"=w501) -> ()  [unwired: 9 in, 1 out]
              }
              frame True {
              }
            }
          }
        }
        n162 = local read "Dest_1"() -> (w404:bool)
        n163 = local read "Dest_3"() -> (w406:bool)
        n164 = local read "Dest_0"() -> (w403:bool)
        n165 = local read "Dest_2"() -> (w405:bool)
        n166 = Build Array(w403, w404, w405, w406) -> (w401:bool[])
        n167 = Or(x=w402, y=w401) -> (x .or. y?=w400:bool[])
        n168 = Or(x=w399, y=w400) -> (x .or. y?=w398:bool[])
      }
    }
  }
  n169 = disable-structure shown="Activé" {
    frame Disabled {
      n170 = local read "Appel_1"() -> (w520:bool)
      n171 = local read "Appel_3"() -> (w522:bool)
      n172 = local read "Appel_0"() -> (w519:bool)
      n173 = local read "Appel_2"() -> (w521:bool)
      n174 = local read "Dest_1"() -> (w525:bool)
      n175 = local read "Dest_3"() -> (w523:bool)
      n176 = local read "Dest_0"() -> (w526:bool)
      n177 = local read "Dest_2"() -> (w524:bool)
      n178 = Build Array(w526, w525, w524, w523) -> (w528:bool[])
      n179 = Build Array(w519, w520, w521, w522) -> (w527:bool[])
      n180 = Or(x=w527, y=w528) -> (x .or. y?=w529:bool[])
      n181 = Or(y=w529) -> ()  [unwired: 1 in, 1 out]
      n182 = local read "P1"() -> (w531:bool)
      n183 = local read "P0"() -> (w530:bool)
      n184 = local read "P2"() -> (w532:bool)
      n185 = local read "P3"() -> (w533:bool)
      n186 = Build Array(w530, w531, w532, w533) -> (w534:bool[])
      n187 = Index Array(array=w534) -> ()  [unwired: 1 in, 1 out]
    }
    frame Enabled {
    }
  }
  n188 = Not(x=w2) -> (.not. x?=w1:bool)
  n189 = local write "Moteur Cabine"(w1) -> ()
  n190 = xnode "myRIO DIO Open.xnode"("Channel Names"=tag[] ["B/DIO0", "B/DIO1"]) -> ("error out"=w4:errorcluster, "DIO Ref Out"=w7:T4)  [unwired: 2 in]
  n191 = call <vilib>:"Write.vi"("error in (no error)"=w4, "Values"=bool[] [TRUE, TRUE], "DIO Ref In"=w7) -> ("error out"=w5:errorcluster, "DIO Ref Out"=w6:T4)  [unwired: 6 in]
  n192 = call <vilib>:"Close.vi"("error in (no error)"=w5, "DIO Ref In"=w6) -> ()  [unwired: 9 in, 1 out]
